vi "DAQ - Init wForms Buffer.vi"(0 "reference in":refnum<class "GSwFormDSP.lvclass">, 5 "error in (no error)":errorcluster) -> (11 "Nb Signals":i32, 13 "DAQ t0":timestamp, 14 "reference out":refnum<class "GSwFormDSP.lvclass">, 19 "error out":errorcluster)   [LabVIEW 2020, in "GSwFormDSP.lvclass"]
uses:
  GSwFormDSP.lvclass
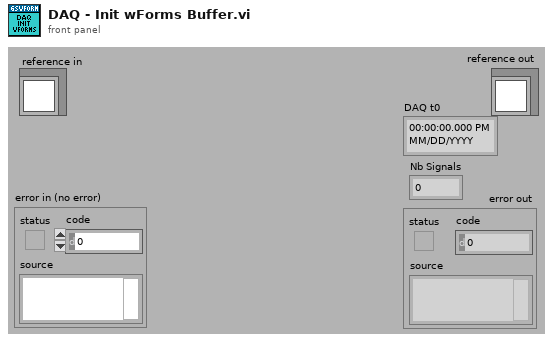
[diagram p1: front panel]
types:
  T1 = typedef "GSwFormDSP.lvclass/ObjectAttributes.ctl" = cluster{"Wform Ref":refnum<data-value>, "Nb Signals":i32, "Spectral Function Parameters":T2, "FFT":waveform(cdb)[], "Nb FFT":i32, "Nb Averages":i32[], "Reference Indexes":i32[], "Response Indexes":i32[], "Coherence":waveform(dbl)[], "TDF Parameters":T4, "DAQ":cluster{"Duration (sec)":dbl, "Buffer Size (Samples)":i32, "Offset (Samples)":i32}, "Filter Impulse Response (TDF)":waveform(dbl), "Sound Playback":T5}
  T2 = typedef "GSwFormDSP.lvclass/Spectral Parameters.ctl" = cluster{"Frequency resolution (Hz)":dbl, "Overlap":dbl, "Window":T3}
  T3 = typedef "NI_AALPro.lvlib/windowTd.ctl" = u32
  T4 = typedef "GSwFormDSP.lvclass/TDF Parameters.ctl" = cluster{"Filter":enum32{"Lowpass", "Highpass", "Bandpass", "Bandstop"}, "Type:":enum16{"Butterworth", "Chebyshev", "Inv Chebyshev", "Elliptic", "Bessel"}, "LP cutoff freq":dbl, "HP cutoff freq":dbl, "Order":i32, "passband ripple (dB)":dbl, "stopband attenuation (dB)":dbl, "Phaseless Filter":bool, "Include Fade IN and OUT":bool}
  T5 = typedef "GSwFormDSP.lvclass/Sound Playback.ctl" = cluster{"Timer start (ms)":u32, "task ID":T6, "Cursor Init Location (s)":dbl, "SC Volume":dbl}
  T6 = typedef "Sound Output Task ID.ctl" = u32
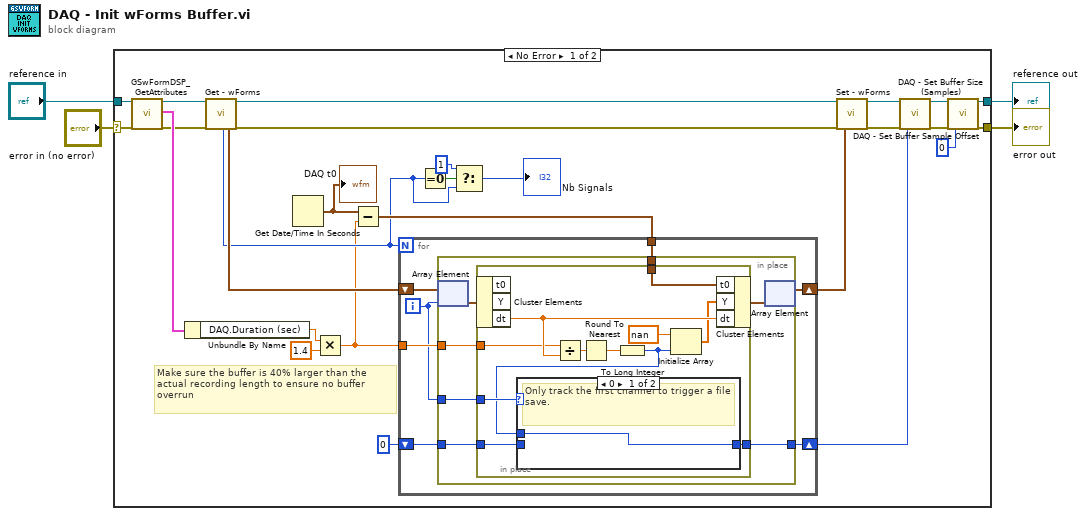
[diagram p0: block diagram]
diagram:
  n1 = case shown="No Error" "error in (no error)" {
    selector: "error in (no error)" -> [w31 w60]
    tunnel: [w6 w60] -> w3
    tunnel: [w7 w59] -> w1
    tunnel: "reference in" -> [w30 w59]
    frame No Error {
      # "Make sure the buffer is 40% larger than the actual recording length to ensure no buffer overrun"
      n2 = call "GSwFormDSP_GetAttributes.vi"("reference in"=w30, "error in (no error)"=w31) -> ("reference out"=w28:refnum<class "GSwFormDSP.lvclass">, "attributes"=w29:T1, "error out"=w27:errorcluster)  [unwired: 14 in, 1 out]
      n3 = Unbundle By Name(w29) -> ("DAQ.Duration (sec)"=w18:dbl)
      n4 = call-dynamic "Get - wForms.vi"("reference in"=w28, "error in (no error)"=w27) -> ("Nb Signals"=w20:i32, "wForms"=w21:waveform(dbl)[], "reference out"=w15:refnum<class "GSwFormDSP.lvclass">, "error out"=w14:errorcluster)  [unwired: 14 in]
      n5 = Get Date/Time In Seconds() -> (seconds since 1Jan1904=w23:timestamp)
      "DAQ t0" <- w23
      n6 = Multiply(x=w18, y=1.4) -> (x*y=w17:dbl)
      n7 = Subtract(x=w23, y=w17) -> (x-y=w22:timestamp)
      n8 = for {
        N: w20 -> [_]
        shift-right: [w37] -> w13
        shift-left: w21 -> [w38]
        tunnel: w17 -> [w36]
        tunnel: w22 -> [w35]
        shift-right: [w33] -> w10
        shift-left: 0 -> [w32]
        i -> [w34]
        n9 = in-place {
          in-place-border: w36 -> [w43]
          in-place-border: w35 -> [w42]
          in-place-border: w34 -> [w41]
          in-place-border: [w40] -> w33
          in-place-border: w32 -> [w39]
          n10 = in-place-array #1(w38, w34) -> (w45:waveform(dbl))
          n11 = in-place {
            in-place-border: w43 -> [w55]
            in-place-border: w42 -> [w50]
            in-place-border: w41 -> [w49]
            in-place-border: [w48] -> w40
            in-place-border: w39 -> [w46]
            n12 = in-place-cluster #2(w45) -> ("dt"=w56:dbl)  [unwired: 2 out]
            n13 = Divide(x=w55, y=w56) -> (x/y=w54:dbl)
            n14 = Round To Nearest(number=w54) -> (nearest integer value=w53:dbl)
            n15 = To Long Integer(number=w53) -> (32bit integer=w47:i32)
            n16 = case shown="0" w49 {
              tunnel: [w57 w58] -> w48
              tunnel: w47 -> [w57 _]
              tunnel: w46 -> [_ w58]
              frame 0 {
                # "Only track the first channel to trigger a file save."
              }
              frame 1, Default {
              }
            }
            n17 = Initialize Array(nan ("element"), w47) -> (w51:dbl[])
            n18 = in-place-cluster #2("t0"=w50, "Y"=w51, "dt"=w56) -> (w44:waveform(dbl))
          }
          n19 = in-place-array #1(w44) -> (w37:waveform(dbl)[])  [unwired: 1 out]
        }
      }
      n20 = Equal To 0?(x=w20) -> (x = 0?=w24:bool)
      n21 = Select(t=1, s=w24, f=w20) -> (s? t:f=→"Nb Signals":i32)
      n22 = call "Set - wForms.vi"("reference in"=w15, "error in (no error)"=w14, "wForms"=w13) -> ("reference out"=w11:refnum<class "GSwFormDSP.lvclass">, "error out"=w12:errorcluster)  [unwired: 15 in]
      n23 = call "DAQ - Set Buffer Size (Samples).vi"("reference in"=w11, "error in (no error)"=w12, "Buffer Size (Samples)"=w10) -> ("reference out"=w9:refnum<class "GSwFormDSP.lvclass">, "error out"=w8:errorcluster)  [unwired: 15 in]
      n24 = call "DAQ - Set Buffer Sample Offset.vi"("reference in"=w9, "error in (no error)"=w8, "DAQ.Offset (Samples)"=0) -> ("reference out"=w7:refnum<class "GSwFormDSP.lvclass">, "error out"=w6:errorcluster)  [unwired: 15 in]
    }
    frame Error {
    }
  }
  "error out" <- w3
  "reference out" <- w1
